vi "Teleop.vi"(10 "Match Info":T1={"Autonomous Elapsed Seconds"=0.0, "TeleOp Elapsed Seconds"=0.0, "Disabled Elapsed Seconds"=0.0, "Visited Autonomous"=FALSE, "Visited TeleOp"=FALSE, "Visited Disabled"=FALSE, "Autonomous Settings"={"Autonomous Style"=enum."Independent", "VI Refnum"=refnum}}, 11 "Call Context":T2) -> ()   [LabVIEW 2011]
doc: "This VI is called for each TeleOp packet received from the DS where the robot is not disabled. It is often used to read from the joysticks and update I/O or to update setpoints for timed control loops. It should complete and return within 20 milliseconds or it may miss DS packets."
uses:
  <vilib>/Rock Robotics/WPI/DriverStation/WPI_DriverStationDerivedRobotMode.ctl
  <vilib>/Rock Robotics/WPI/DriverStation/WPI_DriverStationMatch Info.ctl
  <vilib>/Rock Robotics/WPI/Relay/WPI_RelayValue.ctl
  Robot Global Data.vi
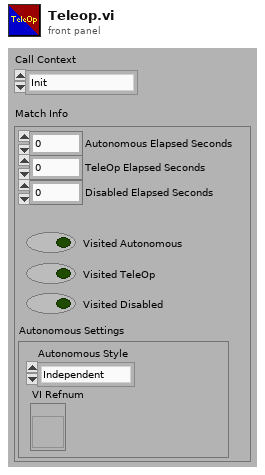
[diagram p1: front panel]
types:
  T1 = typedef "WPI_DriverStationMatch Info.ctl" = cluster{"Autonomous Elapsed Seconds":dbl, "TeleOp Elapsed Seconds":dbl, "Disabled Elapsed Seconds":dbl, "Visited Autonomous":bool, "Visited TeleOp":bool, "Visited Disabled":bool, "Autonomous Settings":cluster{"Autonomous Style":enum16{"Iterative", "Independent"}, "VI Refnum":refnum<vi>}}
  T2 = typedef "WPI_DriverStationDerivedRobotMode.ctl" = enum16{"Init", "Execute", "Stop"}
  T3 = typedef "WPI_RelayValue.ctl" = enum16{"Off", "On", "Forward", "Reverse"}
  T4 = typedef "WPI_JoystickDevRef.ctl" = cluster{"Device":T5}
  T5 = typedef "WPI_JoystickDeviceEnum.ctl" = enum16{"USB 1", "USB 2", "USB 3", "USB 4", "Kinect 1", "Kinect 2"}
  T6 = typedef "WPI_JoystickButtonState.ctl" = cluster{"Button 1":bool, "Button 2":bool, "Button 3":bool, "Button 4":bool, "Button 5":bool, "Button 6":bool, "Button 7":bool, "Button 8":bool, "Button 9":bool, "Button 10":bool, "Button 11":bool, "Button 12":bool}
  T7 = cluster{"axis 1 (x)":dbl, "axis 2 (y)":dbl, "axis 3 (throttle)":dbl, "axis 4":dbl, "axis 5":dbl, "axis 6":dbl}
  T8 = typedef "WPI_MotorControlDeviceRef.ctl" = cluster{"DeviceStatus":errorcluster, "Type":enum16{"PWM", "CAN"}, "PWM":cluster{"Digital Module":T9, "PWM Channel":T10, "DeadBand":T11}, "CAN":cluster{"Device Number":u8, "Control Mode":T12, "Semaphore":T13, "Max Vout":dbl}, "Invert":bool, "TransformRef":T14, "InvTransformRef":T14}
  T9 = typedef "FPGA_TypedefDigitalModule.ctl" = enum16{"Digital Module 1", "Digital Module 2"}
  T10 = typedef "FPGA_DIOPWMChannel.ctl" = enum8{"PWM 1", "PWM 2", "PWM 3", "PWM 4", "PWM 5", "PWM 6", "PWM 7", "PWM 8", "PWM 9", "PWM 10", "Invalid"}
  T11 = typedef "WPI_PWMDeadband.ctl" = cluster{"Name":string, "maxPositivePwm":i32, "minPositivePwm":i32, "centerPwm":i32, "maxNegativePwm":i32, "minNegativePwm":i32, "angularRange":u16}
  T12 = typedef "WPI_CANJaguar_ControlMode.ctl" = enum8{"Percent VBus", "Current", "Speed", "Position", "Voltage"}
  T13 = typedef "Semaphore RefNum" = refnum<k1>
  T14 = typedef "WPI_PWMTransform_ConPane.ctl" = refnum<vi>
  T15 = cluster{"Driver Station Digital Input (1-8)[0]":bool, "Driver Station Digital Input (1-8)[1]":bool, "Driver Station Digital Input (1-8)[2]":bool, "Driver Station Digital Input (1-8)[3]":bool, "Driver Station Digital Input (1-8)[4]":bool, "Driver Station Digital Input (1-8)[5]":bool, "Driver Station Digital Input (1-8)[6]":bool, "Driver Station Digital Input (1-8)[7]":bool, "Driver Station Digital Input (1-8)[8]":bool}
  T16 = typedef "WPI_RelayDevRef.ctl" = cluster{"DevStatus":errorcluster, "Relay Channel":T17, "Digital Module":T9, "Relay Direction":T18}
  T17 = typedef "FPGA_DIORelayChannel.ctl" = enum8{"Relay 1", "Relay 2", "Relay 3", "Relay 4", "Relay 5", "Relay 6", "Relay 7", "Relay 8", "Invalid"}
  T18 = typedef "WPI_RelayDirection.ctl" = enum16{"Both directions", "Forward only", "Reverse only"}
  T19 = typedef "WPI_DigitalInputDevRef.ctl" = cluster{"DevStatus":errorcluster, "DIO Channel":T20, "Digital Module":T9}
  T20 = typedef "FPGA_DIOChannel.ctl" = enum8{"DIO 1", "DIO 2", "DIO 3", "DIO 4", "DIO 5", "DIO 6", "DIO 7", "DIO 8", "DIO 9", "DIO 10", "DIO 11", "DIO 12", "DIO 13", "DIO 14", "Invalid"}
  T21 = typedef "WPI_ServoDeviceRef.ctl" = cluster{"DeviceStatus":errorcluster, "Digital Module":T9, "PWM Channel":T10, "DeadBand":T11}
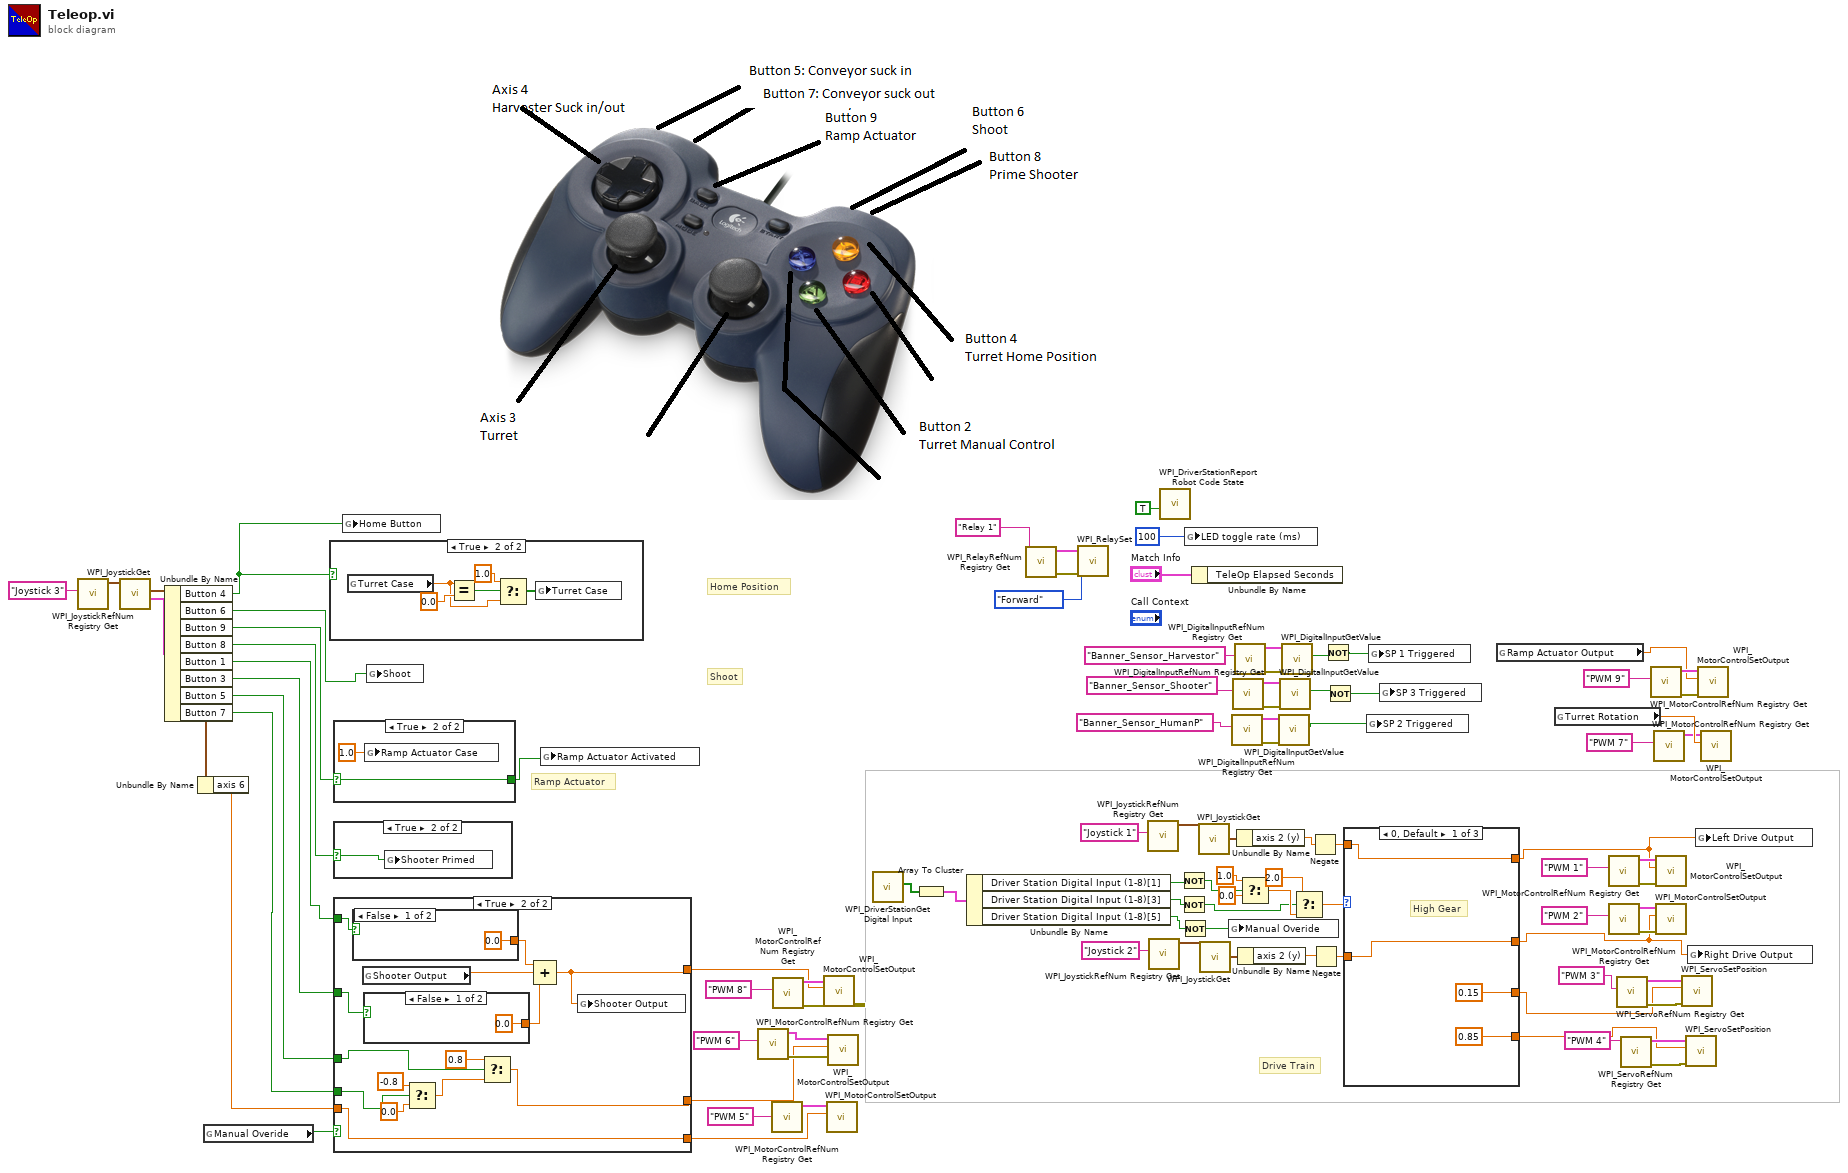
[diagram p0: block diagram]
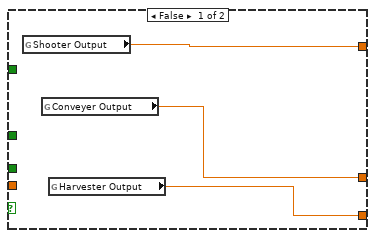
[diagram p2: hidden frame]
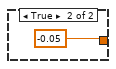
[diagram p3: hidden frame]
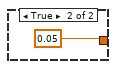
[diagram p4: hidden frame]
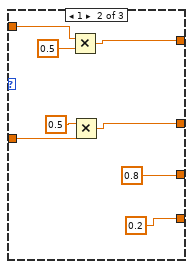
[diagram p8: hidden frame]
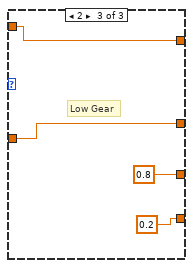
[diagram p9: hidden frame]
diagram:
  # "Home Position"
  # "Shoot"
  # "Ramp Actuator"
  # "Drive Train"
  n1 = call <vilib>:"WPI_JoystickRefNum Registry Get.vi"("refnum name"="Joystick 3") -> ("JoystickDevRef"=w45:T4)  [unwired: 9 in, 1 out]
  n2 = call <vilib>:"WPI_JoystickGet.vi"("JoystickDevRef"=w45) -> ("Buttons"=w46:T6, "Axes"=w17:T7)  [unwired: 4 in, 1 out]
  n3 = Unbundle By Name(w46) -> ("Button 4"=w44:bool, "Button 6"=w43:bool, "Button 9"=w42:bool, "Button 8"=w18:bool, "Button 1"=w12:bool, "Button 3"=w11:bool, "Button 5"=w10:bool, "Button 7"=w9:bool)
  n4 = Unbundle By Name(w17) -> ("axis 6"=w4:dbl)
  n5 = global read "Robot Global Data.vi" "Manual Overide"() -> (w3:bool)
  n6 = case shown="True" w44 {
    frame False {
    }
    frame True {
      n7 = global read "Robot Global Data.vi" "Turret Case"() -> (w95:dbl)
      n8 = Equal?(x=w95, y=0.0) -> (x = y?=w97:bool)
      n9 = Select(t=1.0, s=w97, f=w95) -> (s? t:f=w94:dbl)
      n10 = global write "Robot Global Data.vi" "Turret Case"(w94) -> ()
    }
  }
  n11 = case shown="True" w42 {
    selector: w42 -> [w99 w101]
    tunnel: [w99 w101] -> w48
    frame False {
    }
    frame True {
      n12 = global write "Robot Global Data.vi" "Ramp Actuator Case"(1.0 ("Ramp Actuator Case")) -> ()
    }
  }
  n13 = case shown="True" w18 {
    selector: w18 -> [_ w102]
    frame False {
    }
    frame True {
      n14 = global write "Robot Global Data.vi" "Shooter Primed"(w102) -> ()
    }
  }
  n15 = case shown="True" w3 {
    tunnel: [w105 w106] -> w13
    tunnel: w12 -> [_ w111]
    tunnel: w11 -> [_ w110]
    tunnel: w10 -> [_ w114]
    tunnel: w9 -> [_ w115]
    tunnel: [w103 w113] -> w5
    tunnel: w4 -> [_ w112]
    tunnel: [w104 w112] -> w2
    frame False {
      n16 = global read "Robot Global Data.vi" "Shooter Output"() -> (w105:dbl)
      n17 = global read "Robot Global Data.vi" "Conveyer Output"() -> (w103:dbl)
      n18 = global read "Robot Global Data.vi" "Harvester Output"() -> (w104:dbl)
    }
    frame True {
      n19 = case shown="False" w111 {
        tunnel: [0.0 0.05] -> w109
        frame False {
        }
        frame True {
        }
      }
      n20 = global read "Robot Global Data.vi" "Shooter Output"() -> (w107:dbl)
      n21 = case shown="False" w110 {
        tunnel: [0.0 -0.05] -> w108
        frame False {
        }
        frame True {
        }
      }
      n22 = Select(t=-0.8, s=w115, f=0.0) -> (s? t:f=w119:dbl)
      n23 = Select(t=0.8, s=w114, f=w119) -> (s? t:f=w113:dbl)
      n24 = Compound Arithmetic op=ADD(w109, w107, w108) -> (w106:dbl)
      n25 = global write "Robot Global Data.vi" "Shooter Output"(w106) -> ()
    }
  }
  n26 = global write "Robot Global Data.vi" "Home Button"(w44) -> ()
  n27 = global write "Robot Global Data.vi" "Shoot"(w43) -> ()
  n28 = global write "Robot Global Data.vi" "Ramp Actuator Activated"(w48) -> ()
  n29 = call <vilib>:"WPI_MotorControlRefNum Registry Get.vi"("refnum name"="PWM 6") -> ("error out"=w6:errorcluster, "MotorControlDevRef"=w7:T8)  [unwired: 9 in]
  n30 = call <vilib>:"WPI_MotorControlRefNum Registry Get.vi"("refnum name"="PWM 5") -> ("MotorControlDevRef"=w36:T8)  [unwired: 9 in, 1 out]
  n31 = call <vilib>:"WPI_MotorControlRefNum Registry Get.vi"("refnum name"="PWM 8") -> ("error out"=w20:errorcluster, "MotorControlDevRef"=w21:T8)  [unwired: 9 in]
  n32 = call <vilib>:"WPI_MotorControlSetOutput.vi"("error in (no error)"=w20, "Output"=w13, "MotorControlDevRef"=w21) -> ()  [unwired: 7 in, 2 out]
  n33 = call <vilib>:"WPI_MotorControlSetOutput.vi"("Output"=w2, "MotorControlDevRef"=w36) -> ()  [unwired: 8 in, 2 out]
  n34 = call <vilib>:"WPI_MotorControlSetOutput.vi"("error in (no error)"=w6, "Output"=w5, "MotorControlDevRef"=w7) -> ()  [unwired: 7 in, 2 out]
  n35 = call <vilib>:"WPI_DriverStationGet Digital Input.vi"() -> ("Driver Station Digital Input (1-8)"=w67:bool[])  [unwired: 11 in]
  n36 = Array To Cluster(array=w67) -> (cluster=w90:T15)
  n37 = Unbundle By Name(w90) -> ("Driver Station Digital Input (1-8)[1]"=w70:bool, "Driver Station Digital Input (1-8)[3]"=w69:bool, "Driver Station Digital Input (1-8)[5]"=w14:bool)
  n38 = call <vilib>:"WPI_RelayRefNum Registry Get.vi"("refnum name"="Relay 1") -> ("error out"=w40:errorcluster, "RelayDevRef"=w41:T16)  [unwired: 9 in]
  n39 = call <vilib>:"WPI_RelaySet.vi"("error in (no error)"=w40, "RelayValue"=WPI_RelayValue."Forward", "RelayDevRef"=w41) -> ()  [unwired: 7 in, 2 out]
  n40 = call <vilib>:"WPI_JoystickRefNum Registry Get.vi"("refnum name"="Joystick 1") -> ("JoystickDevRef"=w83:T4)  [unwired: 9 in, 1 out]
  n41 = call <vilib>:"WPI_JoystickRefNum Registry Get.vi"("refnum name"="Joystick 2") -> ("JoystickDevRef"=w80:T4)  [unwired: 9 in, 1 out]
  n42 = call <vilib>:"WPI_DriverStationReport Robot Code State.vi"("TeleOp"=TRUE ("Autonomous")) -> ()  [unwired: 10 in, 1 out]
  n43 = Not(x=w70) -> (.not. x?=w68:bool)
  n44 = Not(x=w69) -> (.not. x?=w16:bool)
  n45 = Not(x=w14) -> (.not. x?=w15:bool)
  n46 = global write "Robot Global Data.vi" "LED toggle rate (ms)"(u32 100 ("LED ms toggle rate")) -> ()
  n47 = Unbundle By Name("Match Info") -> ()  [unwired: 1 out]
  n48 = call <vilib>:"WPI_JoystickGet.vi"("JoystickDevRef"=w83) -> ("Axes"=w82:T7)  [unwired: 4 in, 2 out]
  n49 = call <vilib>:"WPI_JoystickGet.vi"("JoystickDevRef"=w80) -> ("Axes"=w81:T7)  [unwired: 4 in, 2 out]
  n50 = global write "Robot Global Data.vi" "Manual Overide"(w15) -> ()
  n51 = call <vilib>:"WPI_DigitalInputRefNum Registry Get.vi"("refnum name"="Banner_Sensor_HumanP") -> ("error out"=w31:errorcluster, "DigitalInputDevRef"=w30:T19)  [unwired: 9 in]
  n52 = call <vilib>:"WPI_DigitalInputRefNum Registry Get.vi"("refnum name"="Banner_Sensor_Shooter") -> ("error out"=w32:errorcluster, "DigitalInputDevRef"=w33:T19)  [unwired: 9 in]
  n53 = call <vilib>:"WPI_DigitalInputRefNum Registry Get.vi"("refnum name"="Banner_Sensor_Harvestor") -> ("error out"=w35:errorcluster, "DigitalInputDevRef"=w34:T19)  [unwired: 9 in]
  n54 = Unbundle By Name(w82) -> ("axis 2 (y)"=w66:dbl)
  n55 = Unbundle By Name(w81) -> ("axis 2 (y)"=w64:dbl)
  n56 = Select(t=1.0, s=w68, f=0.0 ("t")) -> (s? t:f=w87:dbl)
  n57 = call <vilib>:"WPI_DigitalInputGetValue.vi"("error in (no error)"=w31, "DigitalInputDevRef"=w30) -> ("Value"=w26:bool)  [unwired: 7 in, 2 out]
  n58 = call <vilib>:"WPI_DigitalInputGetValue.vi"("error in (no error)"=w32, "DigitalInputDevRef"=w33) -> ("Value"=w25:bool)  [unwired: 7 in, 2 out]
  n59 = call <vilib>:"WPI_DigitalInputGetValue.vi"("error in (no error)"=w35, "DigitalInputDevRef"=w34) -> ("Value"=w23:bool)  [unwired: 7 in, 2 out]
  n60 = Select(t=2.0, s=w16, f=w87) -> (s? t:f=w85:dbl)
  n61 = Negate(x=w66) -> (-x=w65:dbl)
  n62 = Negate(x=w64) -> (-x=w63:dbl)
  n63 = Not(x=w23) -> (.not. x?=w22:bool)
  n64 = Not(x=w25) -> (.not. x?=w24:bool)
  n65 = case shown="0, Default" w85 {
    tunnel: w63 -> [w127 w132 w139]
    tunnel: [w127 w133 w139] -> w55
    tunnel: [w126 w134 w138] -> w56
    tunnel: [0.15 ("LeftShifter_Pos") 0.8 0.8] -> w72
    tunnel: [0.85 0.2 ("LeftShifter_Pos") 0.2 ("LeftShifter_Pos")] -> w71
    tunnel: w65 -> [w126 w130 w138]
    frame 0, Default {
      # "High Gear"
    }
    frame 1 {
      n66 = Multiply(x=w130, y=0.5) -> (x*y=w134:dbl)
      n67 = Multiply(x=0.5 ("y"), y=w132) -> (x*y=w133:dbl)
    }
    frame 2 {
      # "Low Gear"
    }
  }
  n68 = global write "Robot Global Data.vi" "SP 2 Triggered"(w26) -> ()
  n69 = global write "Robot Global Data.vi" "SP 1 Triggered"(w22) -> ()
  n70 = global write "Robot Global Data.vi" "SP 3 Triggered"(w24) -> ()
  n71 = global read "Robot Global Data.vi" "Ramp Actuator Output"() -> (w1:dbl)
  n72 = global read "Robot Global Data.vi" "Turret Rotation"() -> (w51:dbl)
  n73 = call <vilib>:"WPI_MotorControlRefNum Registry Get.vi"("refnum name"="PWM 1") -> ("error out"=w60:errorcluster, "MotorControlDevRef"=w62:T8)  [unwired: 9 in]
  n74 = call <vilib>:"WPI_MotorControlRefNum Registry Get.vi"("refnum name"="PWM 2") -> ("error out"=w59:errorcluster, "MotorControlDevRef"=w58:T8)  [unwired: 9 in]
  n75 = call <vilib>:"WPI_ServoRefNum Registry Get.vi"("refnum name"="PWM 3") -> ("error out"=w76:errorcluster, "ServoDeviceRef"=w77:T21)  [unwired: 9 in]
  n76 = call <vilib>:"WPI_ServoRefNum Registry Get.vi"("refnum name"="PWM 4") -> ("error out"=w75:errorcluster, "ServoDeviceRef"=w74:T21)  [unwired: 9 in]
  n77 = call <vilib>:"WPI_MotorControlRefNum Registry Get.vi"("refnum name"="PWM 9") -> ("error out"=w53:errorcluster, "MotorControlDevRef"=w52:T8)  [unwired: 9 in]
  n78 = call <vilib>:"WPI_MotorControlRefNum Registry Get.vi"("refnum name"="PWM 7") -> ("MotorControlDevRef"=w49:T8)  [unwired: 9 in, 1 out]
  n79 = call <vilib>:"WPI_MotorControlSetOutput.vi"("error in (no error)"=w60, "Output"=w56, "MotorControlDevRef"=w62) -> ()  [unwired: 7 in, 2 out]
  n80 = call <vilib>:"WPI_MotorControlSetOutput.vi"("error in (no error)"=w59, "Output"=w55, "MotorControlDevRef"=w58) -> ()  [unwired: 7 in, 2 out]
  n81 = call <vilib>:"WPI_ServoSetPosition.vi"("error in (no error)"=w76, "Position"=w72, "ServoDeviceRef"=w77) -> ()  [unwired: 7 in, 2 out]
  n82 = call <vilib>:"WPI_ServoSetPosition.vi"("error in (no error)"=w75, "Position"=w71, "ServoDeviceRef"=w74) -> ()  [unwired: 7 in, 2 out]
  n83 = global write "Robot Global Data.vi" "Right Drive Output"(w55) -> ()
  n84 = global write "Robot Global Data.vi" "Left Drive Output"(w56) -> ()
  n85 = call <vilib>:"WPI_MotorControlSetOutput.vi"("error in (no error)"=w53, "Output"=w1, "MotorControlDevRef"=w52) -> ()  [unwired: 7 in, 2 out]
  n86 = call <vilib>:"WPI_MotorControlSetOutput.vi"("Output"=w51, "MotorControlDevRef"=w49) -> ()  [unwired: 8 in, 2 out]
